vi "Hide Window.vi"(4 "error in (no error)":errorcluster, 6 "window name (\"\")":string, 7 "window refnum (NaWR)":T1) -> (0 "error out":errorcluster, 3 "window refnum out":T1)   [LabVIEW 2023, in "WINUTIL.lvlib"]
doc: "This function will hide the window named in the 'window name' input if 'window refnum' is not valid. Otherwise it uses 'window refnum' to identify the window. If the window cannot be found, an error will be returned. If the winodw name is used to identify the window instead, then 'window refnum out' will contain the window refnum for the window that was hidden if the function was successful."
uses:
  WINUTIL.lvlib
  Window Refnum.ctl
  LVWUtil32.dll
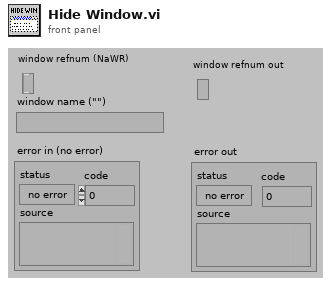
[diagram p1: front panel]
types:
  T1 = typedef "WINUTIL.lvlib/Window Refnum.ctl" = refnum<k1>
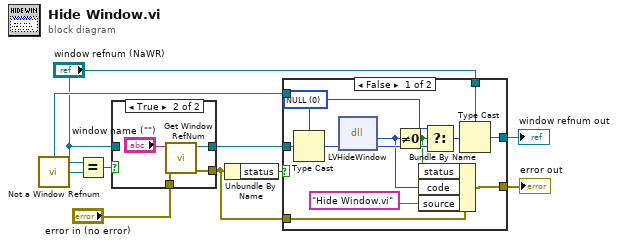
[diagram p0: block diagram]
diagram:
  n1 = call "Not a Window Refnum.vi"() -> ("Not a Window Refnum"=w4:T1)
  n2 = Equal?(x="window refnum (NaWR)", y=w4) -> (x = y?=w5:bool)
  n3 = case shown="True" w5 {
    tunnel: "error in (no error)" -> [w10 w15]
    tunnel: [w11 w14] -> w2
    tunnel: "window refnum (NaWR)" -> [w11 _]
    tunnel: [w10 w13] -> w8
    frame False {
    }
    frame True {
      n4 = call "Get Window RefNum.vi"("error in (no error)"=w15, "window name (\"\")"="window name (\"\")") -> ("error out"=w13:errorcluster, "window refnum (NaWR)"=w14:T1)  [unwired: 6 out]
    }
  }
  n5 = Unbundle By Name(w8) -> ("status"=w9:bool)
  n6 = case shown="False" w9 {
    tunnel: w8 -> [w21 w29]
    tunnel: [w26 w29] -> w6
    tunnel: w2 -> [w18 _]
    tunnel: [w17 w28] -> w1
    tunnel: "window refnum (NaWR)" -> [w16 _]
    tunnel: w4 -> [_ w28]
    frame False {
      w20 = u32 0 items=["NULL"]
      n7 = Type Cast(type=w20, x=w18) -> (*(type *) &x=w19:u32)
      n8 = dll-call lib="C:/Users/acasalen/Documents/LabVIEW Data/Projects/Reds-Auto-Clicker/Red's Auto Clicker/SubVIs/labview_win_util32_8.6/lvwutil32.dll" fn="LVHideWindow"("hWnd"=w19) -> ("error"=w24:i32, "hWnd"=w27:u32)  [unwired: 3 in, 2 out]
      n9 = Not Equal To 0?(x=w24) -> (x != 0?=w23:bool)
      n10 = Bundle By Name(cluster=w21, "status"=w23, "code"=w24, "source"="Hide Window.vi") -> (w26:errorcluster)
      n11 = Select(t=w20, s=w23, f=w27) -> (s? t:f=w25:u32)
      n12 = Type Cast(type=w16, x=w25) -> (*(type *) &x=w17:T1)
    }
    frame True {
    }
  }
  "error out" <- w6
  "window refnum out" <- w1
